vi "Order By Module.vi"(7 "Mode":T1=enum."Request", 11 "Functions":string[](array[string])) -> (3 "Functions by Module":T2[](array[typedef]))   [LabVIEW 2021, in "TAF Proj Document Type.lvlib" / "Project Parser.lvlib"]
uses:
  <vilib>/Wovalab/AntiDoc/Document Type/Add-ons/LabVIEW TAF Project/Project Parser/Project Parser.lvlib
  <vilib>/Wovalab/AntiDoc/Document Type/Add-ons/LabVIEW TAF Project/Project Parser/Module Fonctions--cluster.ctl
  <vilib>/Wovalab/AntiDoc/Document Type/Add-ons/LabVIEW TAF Project/Project Parser/Module Fonctions--enum.ctl
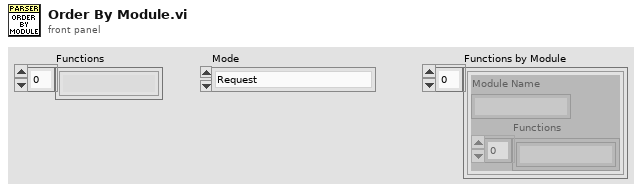
[diagram p1: front panel]
types:
  T1 = typedef "TAF Proj Document Type.lvlib/Project Parser.lvlib/Module Fonctions--enum.ctl" = enum16{"Event Registration", "Request"}
  T2 = typedef "TAF Proj Document Type.lvlib/Project Parser.lvlib/Module Fonctions--cluster.ctl" = cluster{"Module Name":string, "Functions":string[]}
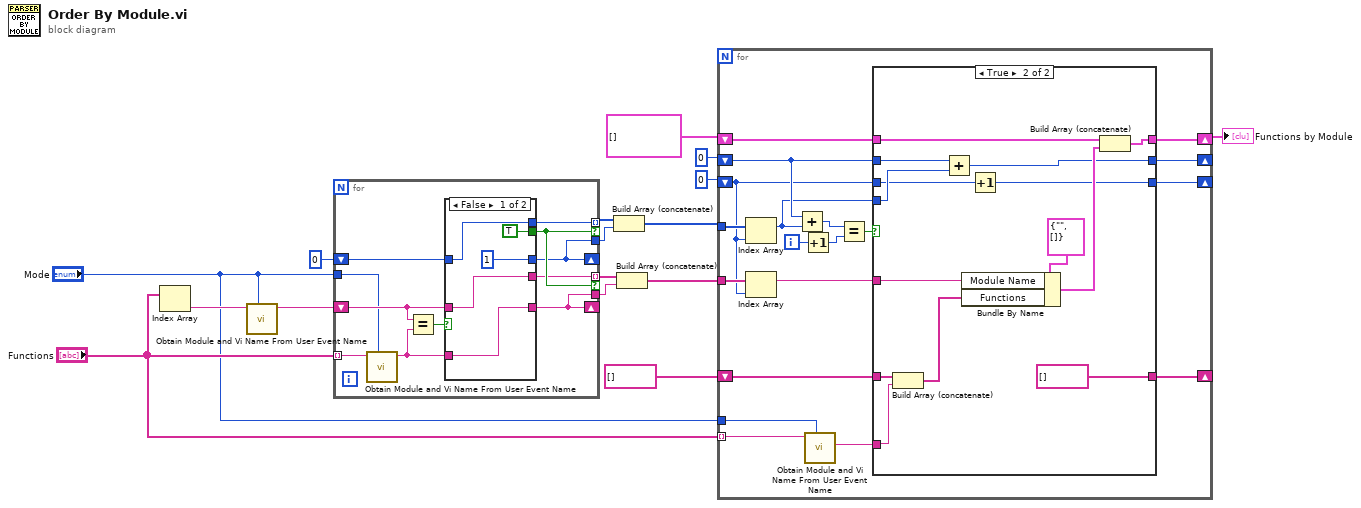
[diagram p0: block diagram]
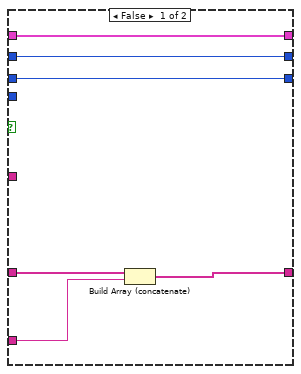
[diagram p2: hidden frame]
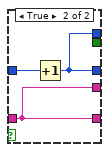
[diagram p3: hidden frame]
diagram:
  n1 = Index Array(array="Functions") -> (element=w2:string)  [unwired: 1 in]
  n2 = call <vilib>:"Obtain Module and Vi Name From User Event Name.vi"("Mode"="Mode", "User Event Name"=w2) -> ("Module"=w3:string)  [unwired: 8 in, 1 out]
  n3 = for {
    tunnel: "Functions" -> [w25] mode=indexing
    shift-right: [w18] -> _
    shift-left: w3 -> [w26]
    shift-right: [w19] -> _
    shift-left: 0 -> [w27]
    tunnel: [w21] -> w5 mode=indexing if=w23
    tunnel: [w20] -> w8 mode=indexing if=w23
    tunnel: [w19] -> w6
    tunnel: [w18] -> w7
    tunnel: "Mode" -> [w17]
    n4 = call <vilib>:"Obtain Module and Vi Name From User Event Name.vi"("Mode"=w17, "User Event Name"=w25) -> ("Module"=w24:string)  [unwired: 8 in, 1 out]
    n5 = Equal?(x=w26, y=w24) -> (x = y?=w22:bool)
    n6 = case shown="False" w22 {
      tunnel: w27 -> [w32 w35]
      tunnel: [1 w33] -> w19
      tunnel: [w32 w33] -> w21
      tunnel: [w28 w34] -> w18
      tunnel: w24 -> [w28 _]
      tunnel: w26 -> [w29 w34]
      tunnel: [w29 w34] -> w20
      tunnel: [TRUE _] -> w23
      frame False {
      }
      frame True {
        n7 = Increment(x=w35) -> (x+1=w33:i32)
      }
    }
  }
  n8 = Build Array (concatenate)(w5, w6) -> (w11:i32[])
  n9 = Build Array (concatenate)(w8, w7) -> (w10:string[])
  n10 = for {
    tunnel: "Functions" -> [w54] mode=indexing
    tunnel: w10 -> [w48]
    tunnel: w11 -> [w52]
    shift-right: [w49] -> w13
    shift-left: T2[] [] ("Registred Broadcast") -> [w50]
    shift-right: [w45] -> _
    shift-left: string[] [] ("appended array") -> [w46]
    shift-right: [w43] -> _
    shift-left: 0 -> [w41]
    shift-right: [w38] -> _
    shift-left: 0 -> [w39]
    tunnel: "Mode" -> [w36]
    i -> [w53]
    n11 = Index Array(array=w52, index=w39) -> (element=w37:i32)
    n12 = Index Array(array=w48, index=w39) -> (element=w40:string)
    n13 = Add(x=w41, y=w37) -> (x+y=w42:i32)
    n14 = Increment(x=w53) -> (x+1=w44:i32)
    n15 = call <vilib>:"Obtain Module and Vi Name From User Event Name.vi"("Mode"=w36, "User Event Name"=w54) -> ("Vi"=w47:string)  [unwired: 8 in, 1 out]
    n16 = Equal?(x=w42, y=w44) -> (x = y?=w51:bool)
    n17 = case shown="True" w51 {
      tunnel: w50 -> [w60 w72]
      tunnel: [w60 w71] -> w49
      tunnel: w40 -> [_ w70]
      tunnel: w47 -> [w59 w68]
      tunnel: w46 -> [w58 w69]
      tunnel: [w57 string[] []] -> w45
      tunnel: w37 -> [_ w65]
      tunnel: w41 -> [w56 w64]
      tunnel: [w56 w63] -> w43
      tunnel: w39 -> [w55 w62]
      tunnel: [w55 w61] -> w38
      frame False {
        n18 = Build Array (concatenate)(w58, w59) -> (w57:string[])
      }
      frame True {
        n19 = Build Array (concatenate)(w69, w68) -> (w67:string[])
        n20 = Add(x=w64, y=w65) -> (x+y=w63:i32)
        n21 = Bundle By Name(cluster=T2 {"Module Name"="", "Functions"=[]} ("Module Broadcast Registred"), "Module Name"=w70, "Functions"=w67) -> (w73:T2)
        n22 = Increment(x=w62) -> (x+1=w61:i32)
        n23 = Build Array (concatenate)(w72, w73) -> (w71:T2[])
      }
    }
  }
  "Functions by Module" <- w13
